vi "Read Liquid Level.vi"(8 "error in":errorcluster, 11 "CPC in":refnum<class "CPC.lvclass">) -> (0 "error out":errorcluster, 2 "Liquid Level":T1, 3 "CPC out":refnum<class "CPC.lvclass">)   [LabVIEW 2013, in "CPC.lvclass"]
uses:
  CPC.lvclass
  Controls/Liquid Level.ctl
  CPC.lvclass/CPC.ctl
  Reusable/Session APIs/Serial/Public/Get Data/Get String.vi
  Reusable/Session APIs/Serial/Serial Session.lvclass
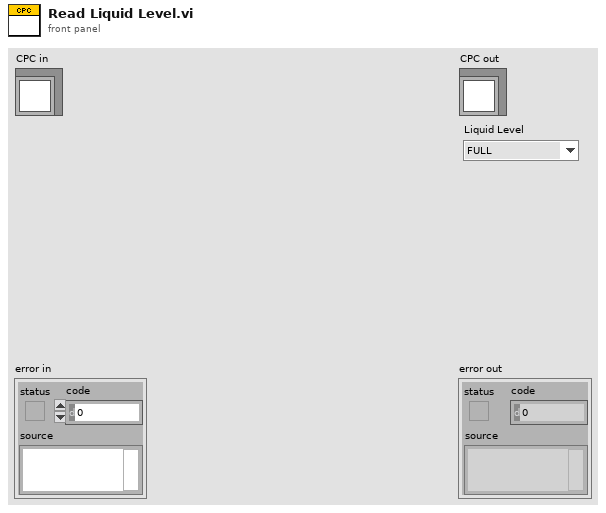
[diagram p1: front panel]
types:
  T1 = typedef "CPC.lvclass/Liquid Level.ctl" = enum16{"FULL", "NOTFULL"}
  T2 = typedef "Serial Session.lvclass/Session Handle.ctl" = refnum<data-value>
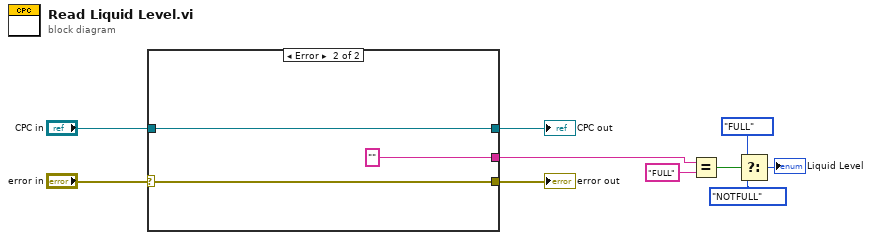
[diagram p0: block diagram]
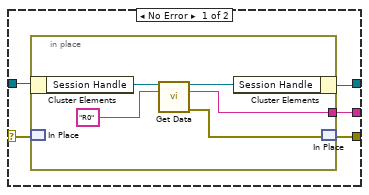
[diagram p2: hidden frame]
diagram:
  n1 = case shown="Error" "error in" {
    selector: "error in" -> [w14 w23]
    tunnel: "CPC in" -> [w15 w22]
    tunnel: [w12 w23] -> w2
    tunnel: [w13 w22] -> w3
    tunnel: [w11 "" ("DataOut")] -> w4
    frame No Error {
      n2 = in-place {
        in-place-border: [w17] -> w11
        n3 = in-place-cluster #1(w15) -> ("Session Handle"=w20:T2)
        n4 = in-place-match #2(w14) -> ()  [unwired: 1 out]
        n5 = call-poly "Get Data.vi"("Session Handle in"=w20, "CMD"="R0" ("string")) -> ("Session Handle out"=w19:T2, "DataOut"=w17:string, "error out"=w18:errorcluster)  [unwired: 11 in]
        n6 = in-place-cluster #1("Session Handle"=w19) -> (w13:refnum<class "CPC.lvclass">)
        n7 = in-place-match #2(w18) -> (w12:errorcluster)
      }
    }
    frame Error {
    }
  }
  "error out" <- w2
  "CPC out" <- w3
  n8 = Equal?(x=w4, y="FULL") -> (x = y?=w8:bool)
  n9 = Select(t=Liquid_Level."FULL" ("Liquid Level"), s=w8, f=Liquid_Level."NOTFULL" ("Liquid Level")) -> (s? t:f=→"Liquid Level":T1)
